vi "Soft_Robot_Model.vi"() -> ()   [LabVIEW 2015]
uses:
  <vilib>/addons/Control Design/_Stochastic Systems/Stochastic Systems.llb/Stochastic Systems SubVIs/cd_Stochastic State-Space Model.ctl
  <vilib>/addons/Control Design/_Model Construction/Model Typedefs.llb/CD State Space Model (MIMO).ctl
  <vilib>/addons/Control Design/_Model Construction/Model Typedefs.llb/CD General Elements.ctl
  <vilib>/addons/Control Design/_Stochastic Systems/Stochastic Systems.llb/Stochastic Systems SubVIs/cd_Second-Order Statistics Noise Model.ctl
  <vilib>/Analysis/Matrix/Datatypes/RealMatrix.ctl
  <vilib>/addons/Control Design/_Stochastic Systems/Stochastic Systems.llb/CD CtoD Stochastic Model.ctl
  <vilib>/Analysis/7linalg.llb/Eigenvalue and Vectors Output Option.ctl
  <vilib>/Platform/TimedLoop/XDataNode/timing_clust.ctl
  <vilib>/Platform/TimedLoop/XDataNode/nitl_modes.ctl
  <vilib>/Platform/TimedLoop/XDataNode/wakeup.ctl
  <vilib>/addons/Control Design/_Stochastic Systems/Stochastic Systems.llb/CD Construct Stochastic Model (Numeric).vi
  <vilib>/Analysis/7linalg.llb/Create Special Real Matrix.vi
  <vilib>/addons/Control Design/_Stochastic Systems/Stochastic Systems.llb/CD Construct Noise Model (Numeric).vi
  <vilib>/Analysis/7linalg.llb/Real Eigenvalues and Vectors.vi
  <vilib>/addons/Control Design/_State Feedback Control/State Feedback Control.llb/State Feedback Control SubVis/cd_Linear Quadratic Regulator.vi
  <vilib>/FPGAPlugInAG/myRIO-1900/niLvFpga_Open_myRIO-1900.vi
  <vilib>/rvi/interface/common/dynamic/niFpgaDynamicAddResources.vi
  <vilib>/Utility/error.llb/Error Cluster From Error Code.vi
  <vilib>/rvi/errors/niLvFpgaAdjustHostInterfaceError.vi
  <vilib>/FPGAPlugInAG/Dynamic/niLvFpga_Close_Dynamic.vi
  <vilib>/Utility/file.llb/Write Delimited Spreadsheet (DBL).vi
  <vilib>/Utility/file.llb/Write Delimited Spreadsheet (I64).vi
  <vilib>/addons/Control Design/_Time Response Analysis/Time Response.llb/Time Response subVI/cd_Impulse Response (State-Space).vi
  <vilib>/addons/Control Design/_Time Response Analysis/Time Response.llb/Time Response subVI/cd_Step Response (State-Space).vi
  <vilib>/Simulation/Estimation/Implementation/NILVSim Discrete Kalman Filter.llb/SIM Disc KF Pred and Corr with Pred Gain with Checking Direct LV.vi
  <vilib>/addons/Control Design/_Implementation/CD State Feedback Controller (Multiple Outputs).vi
  <vilib>/Platform/TimedLoop/XDataNode/XDataNode.xnode
  <vilib>/rvi/interface/nirviOpenFPGA/nirviOpenFPGA.xnode
  FPGA Bitfiles/ACC20115_FPGATarget_CurrentControlle_W-6n2rsGK8k.lvbitx
  Misc/Current Controller.vi
  <vilib>/rvi/interface/nirviReadWriteControl/nirviReadWriteControl.xnode
  <vilib>/rvi/interface/nirviCloseFPGA/nirviCloseFPGA.xnode
  <vilib>/Simulation/Implementation/XNodeFramework/SimXNode/SimX.xnode
  <vilib>/addons/Control Design/_State Feedback Control/NI_CD_State Feedback Control.lvlib
  <vilib>/Analysis/NI_AALPro.lvlib
  <vilib>/Platform/TimedLoop/XDataNode/XDNodeRunTimeDep.lvlib
  <vilib>/rvi/interface/Simulation/niFpgaSimulationCallBeginRW.vi
  <vilib>/addons/Control Design/_Stochastic Systems/NI_CD_Stochastic Systems.lvlib
  <vilib>/addons/Control Design/_State-Space Analysis/NI_CD_State-Space Analysis.lvlib
  <vilib>/addons/Control Design/_Implementation/NI_CD_Implementation.lvlib
  <vilib>/addons/Control Design/_Time Response Analysis/NI_CD_Time Response.lvlib
  NiFpgaLv.dll
  <vilib>/addons/Control Design/_Model Construction/NI_LinSys_Model Typedefs.lvlib
  <vilib>/Analysis/Matrix/NI_Matrix.lvlib
panel:
  in  "Tab Control":T1(tab)
  out "Valve Current (mA)":dbl(graph)=181.17310975569308
  out "Kinect Fusion":dbl(graph)=696.694
  in  "Current (mA)":i32
  out "KF Xhat(k|k)":dbl[][](graph)
  out "Plant Output and KF estimation":dbl[][](graph)=[[694.135, 693.2125685090368]]
  out "KF Predictor Gain L(k)":dbl[][](array[numeric])=[[1.0]] format="%#.6g"
  out "KF Gain M(k)":dbl[][](array[numeric]) format="%#.6g"
  in  "Stop":bool
  out "LQR Eigenvalues":cdb[](array[numeric]) format="%.5f"
  out "P(k+1|k)":dbl[][](array[numeric])
  out "P(k|k)":dbl[][](array[numeric])
  out "LQR Q Eig Vals":cdb[](array[numeric])
  out "LQR R Eig Val":cdb[](array[numeric])
  out "Optimal LQR Gains":dbl[][](array[numeric])
  out "Control Action":dbl
  out "Controllable?":bool
  out "Stable?":bool
  out "Detectable?":bool
  out "Observable?":bool
  out "LQR Q Matrix":T2
  out "LQR R Matrix":T2
  out "FPGA Overflow?":bool
  in  "Set Point (mm)":dbl(knob)=641.7660208643815 scale=680.0..700.0
  out "Stochastic SS Model":T3={"Sampling Time (s)"=0.0, "G"=[], "B"=[[-1.71e-07], [6.47e-07]], "A"=[], "C"=[], "D"=[], "H"=[]} {"H" format="%#.2g"; "D" format="%#.2g"; "C" format="%#.2g"; "A" format="%#.2g"; "B" format="%#.2g"; "G" format="%#.2g"; "Sampling Time (s)" format="%.2f"}
  out "Deterministic SS Model":T4={"properties"={"Model name"="", "Input names"=[], "Output names"=[], "Input Delays"=[], "Output Delays"=[], "Sampling Time"=0.0, "Notes"=""}, "A"=[], "B"=[[-1.706e-07], [6.469e-07]], "C"=[], "D"=[], "StateNames"=[], "Transport Delay"=[]} {"Transport Delay" format="%.2f"; "D" format="%#.2g"; "C" format="%#.2g"; "B" format="%#.2g"; "A" format="%#.2g"; "properties"."Sampling Time" format="%#.6p"; "properties"."Output Delays" format="%.4f"; "properties"."Input Delays" format="%.4f"}
  out "DAC Loop Error":errorcluster
  out "LQR Error":errorcluster
  out "KF Noise Model":T6 {"N" format="%#.2g"; "R" format="%#.2g"; "E{v}" format="%#.2g"; "E{w}" format="%#.2g"; "Q" format="%#.2g"}
  out "FPGA Loop Error":errorcluster
  out "Control Loop Error":errorcluster
  out "KF Model Error":errorcluster
  out "UDP Loop Error":errorcluster
  out "Step Response Graph":cluster{"time":dbl[], dbl[]}[](graph)=[{"time"=[0.0, 0.1, 0.2, 0.30000000000000004, 0.4, 0.5, 0.6000000000000001, 0.7000000000000001, 0.8, 0.9, 1.0, 1.1, 1.2000000000000002, 1.3, 1.4000000000000001, 1.5, 1.6, 1.7000000000000002, 1.8, 1.9000000000000001, 2.0, 2.1, 2.2, 2.3000000000000003, 2.4000000000000004, 2.5, 2.6, 2.7, 2.8000000000000003, 2.9000000000000004, 3.0, 3.1, 3.2, 3.3000000000000003, 3.4000000000000004, 3.5, 3.6, 3.7, 3.8000000000000003, 3.9000000000000004, 4.0, 4.1000000000000005, 4.2, 4.3, 4.4, 4.5, 4.6000000000000005, 4.7, 4.800000000000001, 4.9, 5.0, 5.1000000000000005, 5.2, 5.300000000000001, 5.4, 5.5, 5.6000000000000005, 5.7, 5.800000000000001, 5.9, 6.0, 6.1000000000000005, 6.2, 6.300000000000001, 6.4, 6.5, 6.6000000000000005, 6.7, 6.800000000000001, 6.9, 7.0, 7.1000000000000005, 7.2, 7.300000000000001, 7.4, 7.5, 7.6000000000000005, 7.7, 7.800000000000001, 7.9, 8.0], [0.0, 0.0004663473208612627, 0.0017296930483795164, 0.0035885524413313812, 0.00585108885158747, 0.008342022204108804, 0.010907538001557412, 0.013418337758795643, 0.01577103010603519, 0.017888100567384182, 0.019716719021094366, 0.02122664935211373, 0.022407518377011763, 0.02326568343598631, 0.02382091276348735, 0.024103062386256875, 0.024148900146291487, 0.023999193507947617, 0.02369614475738421, 0.023281226369499006, 0.02279344169187109, 0.022268012342287972, 0.021735474206151545, 0.021221148763839872, 0.020744945570676618, 0.020321444775591793, 0.01996020519209235, 0.019666243132932183, 0.01944062944497821, 0.019281156374667745, 0.019183031510994153, 0.01913956258079366, 0.019142803850451515, 0.019184141922185993, 0.01925480547445023, 0.01934628972900578, 0.019450691946355205, 0.019560958936806403, 0.019671051366119408, 0.01977603252338114, 0.019872091237783975, 0.01995650984687708, 0.020027588622327185, 0.02008453795668775, 0.020127349020610013, 0.02015665263024424, 0.020173574831124263, 0.02017959631108057, 0.02017642129264157, 0.02016586010332895, 0.020149728243942358, 0.02012976351919565, 0.020107561696361465, 0.0200845302370225, 0.0200618589138676, 0.02004050557782586, 0.020021194971562285, 0.020004428277976674, 0.01999050102686616, 0.019979527036564866, 0.0199714662161444, 0.019966154273690646, 0.019963332644441115, 0.019962677248304108, 0.019963824991160707, 0.019966397222957007, 0.019970019645588307, 0.019974338415697335, 0.019979032405429503, 0.019983821764274674, 0.01998847306610796, 0.01999280142814749, 0.019996670055101227, 0.019999987695808956, 0.020002704505559007, 0.020004806789810977, 0.02000631106930135, 0.020007257857379883, 0.020007705482562522, 0.0200077242268862, 0.02000739098734998]}]
  out "Impulse Response":cluster{"time":dbl[], dbl[]}[](graph)=[{"time"=[0.0, 0.1, 0.2, 0.30000000000000004, 0.4, 0.5, 0.6000000000000001, 0.7000000000000001, 0.8, 0.9, 1.0, 1.1, 1.2000000000000002, 1.3, 1.4000000000000001, 1.5, 1.6, 1.7000000000000002, 1.8, 1.9000000000000001, 2.0, 2.1, 2.2, 2.3000000000000003, 2.4000000000000004, 2.5, 2.6, 2.7, 2.8000000000000003, 2.9000000000000004, 3.0, 3.1, 3.2, 3.3000000000000003, 3.4000000000000004, 3.5, 3.6, 3.7, 3.8000000000000003, 3.9000000000000004, 4.0, 4.1000000000000005, 4.2, 4.3, 4.4, 4.5, 4.6000000000000005, 4.7, 4.800000000000001, 4.9, 5.0, 5.1000000000000005, 5.2, 5.300000000000001, 5.4, 5.5, 5.6000000000000005, 5.7, 5.800000000000001, 5.9, 6.0, 6.1000000000000005, 6.2, 6.300000000000001, 6.4, 6.5, 6.6000000000000005, 6.7, 6.800000000000001, 6.9, 7.0, 7.1000000000000005, 7.2, 7.300000000000001, 7.4, 7.5, 7.6000000000000005, 7.7, 7.800000000000001, 7.9, 8.0], [0.0, 0.008988172215977587, 0.015941438633037666, 0.02091487162309135, 0.024042908393783827, 0.02551889757722494, 0.02557569478365717, 0.024467992676866855, 0.022456868580669295, 0.019796844996257237, 0.016725591461953054, 0.013456253705261323, 0.010172280017081137, 0.007024525658691236, 0.004130353039235721, 0.0015744064999214857, -0.0005892768149515742, -0.002334157452931432, -0.0036574068645988137, -0.004575736995437892, -0.005121104002831364, -0.005336502802076594, -0.005272025764550862, -0.004981315552097141, -0.004518500722641401, -0.003935664888301879, -0.0032808669235171064, -0.0025967016806585676, -0.001919368189106927, -0.0012781953978247278, -0.0006955639255905182, -0.0001871555662120171, 0.0002375401230830873, 0.0005745316131444697, 0.0008245089129275849, 0.0009919638112413014, 0.0010842980213564997, 0.0011109616697939839, 0.0010826555079039139, 0.0010106212985917036, 0.0009060364188353945, 0.0007795211078167689, 0.000640760178844977, 0.0004982355180431294, 0.00035906135961267507, 0.00022891114129368586, 0.0001120226402826769, 1.1266967989904443e-05, -7.17332656671379e-05, -0.00013645086398689086, -0.0001832792705777772, -0.0002133479298936649, -0.00022833790229576505, -0.0002303060085980187, -0.00022152389413133484, -0.00020433657074322872, -0.00018104328983030286, -0.0001538020745465803, -0.00012455793086593947, -9.499368500849999e-05, -6.650156442132397e-05, -4.0173044664881016e-05, -1.6804109357439747e-05, 3.087108111676786e-06, 1.9233341685522883e-05, 3.158477953815003e-05, 4.027189426429472e-05, 4.556687476968165e-05, 4.7845653868121716e-05, 4.755213725597536e-05, 4.516584913005334e-05, 4.117383523520003e-05, 3.6047319585871326e-05, 3.0223306623967816e-05, 2.4091062632339335e-05, 1.7983202024296476e-05, 1.2170946052935176e-05, 6.863011578249593e-06, 2.207522022942255e-06, -1.7036935523276584e-06, -4.8290401595337954e-06]}]
  out "Step and Impulse Response Plots":cluster{"time":dbl[], dbl[]}[](graph)=[{"time"=[0.0, 0.1, 0.2, 0.30000000000000004, 0.4, 0.5, 0.6000000000000001, 0.7000000000000001, 0.8, 0.9, 1.0, 1.1, 1.2000000000000002, 1.3, 1.4000000000000001, 1.5, 1.6, 1.7000000000000002, 1.8, 1.9000000000000001, 2.0, 2.1, 2.2, 2.3000000000000003, 2.4000000000000004, 2.5, 2.6, 2.7, 2.8000000000000003, 2.9000000000000004, 3.0, 3.1, 3.2, 3.3000000000000003, 3.4000000000000004, 3.5, 3.6, 3.7, 3.8000000000000003, 3.9000000000000004, 4.0, 4.1000000000000005, 4.2, 4.3, 4.4, 4.5, 4.6000000000000005, 4.7, 4.800000000000001, 4.9, 5.0, 5.1000000000000005, 5.2, 5.300000000000001, 5.4, 5.5, 5.6000000000000005, 5.7, 5.800000000000001, 5.9, 6.0, 6.1000000000000005, 6.2, 6.300000000000001, 6.4, 6.5, 6.6000000000000005, 6.7, 6.800000000000001, 6.9, 7.0, 7.1000000000000005, 7.2, 7.300000000000001, 7.4, 7.5, 7.6000000000000005, 7.7, 7.800000000000001, 7.9, 8.0], [0.0, 0.0004663473208612627, 0.0017296930483795164, 0.0035885524413313812, 0.00585108885158747, 0.008342022204108804, 0.010907538001557412, 0.013418337758795643, 0.01577103010603519, 0.017888100567384182, 0.019716719021094366, 0.02122664935211373, 0.022407518377011763, 0.02326568343598631, 0.02382091276348735, 0.024103062386256875, 0.024148900146291487, 0.023999193507947617, 0.02369614475738421, 0.023281226369499006, 0.02279344169187109, 0.022268012342287972, 0.021735474206151545, 0.021221148763839872, 0.020744945570676618, 0.020321444775591793, 0.01996020519209235, 0.019666243132932183, 0.01944062944497821, 0.019281156374667745, 0.019183031510994153, 0.01913956258079366, 0.019142803850451515, 0.019184141922185993, 0.01925480547445023, 0.01934628972900578, 0.019450691946355205, 0.019560958936806403, 0.019671051366119408, 0.01977603252338114, 0.019872091237783975, 0.01995650984687708, 0.020027588622327185, 0.02008453795668775, 0.020127349020610013, 0.02015665263024424, 0.020173574831124263, 0.02017959631108057, 0.02017642129264157, 0.02016586010332895, 0.020149728243942358, 0.02012976351919565, 0.020107561696361465, 0.0200845302370225, 0.0200618589138676, 0.02004050557782586, 0.020021194971562285, 0.020004428277976674, 0.01999050102686616, 0.019979527036564866, 0.0199714662161444, 0.019966154273690646, 0.019963332644441115, 0.019962677248304108, 0.019963824991160707, 0.019966397222957007, 0.019970019645588307, 0.019974338415697335, 0.019979032405429503, 0.019983821764274674, 0.01998847306610796, 0.01999280142814749, 0.019996670055101227, 0.019999987695808956, 0.020002704505559007, 0.020004806789810977, 0.02000631106930135, 0.020007257857379883, 0.020007705482562522, 0.0200077242268862, 0.02000739098734998]}, {"time"=[0.0, 0.1, 0.2, 0.30000000000000004, 0.4, 0.5, 0.6000000000000001, 0.7000000000000001, 0.8, 0.9, 1.0, 1.1, 1.2000000000000002, 1.3, 1.4000000000000001, 1.5, 1.6, 1.7000000000000002, 1.8, 1.9000000000000001, 2.0, 2.1, 2.2, 2.3000000000000003, 2.4000000000000004, 2.5, 2.6, 2.7, 2.8000000000000003, 2.9000000000000004, 3.0, 3.1, 3.2, 3.3000000000000003, 3.4000000000000004, 3.5, 3.6, 3.7, 3.8000000000000003, 3.9000000000000004, 4.0, 4.1000000000000005, 4.2, 4.3, 4.4, 4.5, 4.6000000000000005, 4.7, 4.800000000000001, 4.9, 5.0, 5.1000000000000005, 5.2, 5.300000000000001, 5.4, 5.5, 5.6000000000000005, 5.7, 5.800000000000001, 5.9, 6.0, 6.1000000000000005, 6.2, 6.300000000000001, 6.4, 6.5, 6.6000000000000005, 6.7, 6.800000000000001, 6.9, 7.0, 7.1000000000000005, 7.2, 7.300000000000001, 7.4, 7.5, 7.6000000000000005, 7.7, 7.800000000000001, 7.9, 8.0], [0.0, 0.008988172215977587, 0.015941438633037666, 0.02091487162309135, 0.024042908393783827, 0.02551889757722494, 0.02557569478365717, 0.024467992676866855, 0.022456868580669295, 0.019796844996257237, 0.016725591461953054, 0.013456253705261323, 0.010172280017081137, 0.007024525658691236, 0.004130353039235721, 0.0015744064999214857, -0.0005892768149515742, -0.002334157452931432, -0.0036574068645988137, -0.004575736995437892, -0.005121104002831364, -0.005336502802076594, -0.005272025764550862, -0.004981315552097141, -0.004518500722641401, -0.003935664888301879, -0.0032808669235171064, -0.0025967016806585676, -0.001919368189106927, -0.0012781953978247278, -0.0006955639255905182, -0.0001871555662120171, 0.0002375401230830873, 0.0005745316131444697, 0.0008245089129275849, 0.0009919638112413014, 0.0010842980213564997, 0.0011109616697939839, 0.0010826555079039139, 0.0010106212985917036, 0.0009060364188353945, 0.0007795211078167689, 0.000640760178844977, 0.0004982355180431294, 0.00035906135961267507, 0.00022891114129368586, 0.0001120226402826769, 1.1266967989904443e-05, -7.17332656671379e-05, -0.00013645086398689086, -0.0001832792705777772, -0.0002133479298936649, -0.00022833790229576505, -0.0002303060085980187, -0.00022152389413133484, -0.00020433657074322872, -0.00018104328983030286, -0.0001538020745465803, -0.00012455793086593947, -9.499368500849999e-05, -6.650156442132397e-05, -4.0173044664881016e-05, -1.6804109357439747e-05, 3.087108111676786e-06, 1.9233341685522883e-05, 3.158477953815003e-05, 4.027189426429472e-05, 4.556687476968165e-05, 4.7845653868121716e-05, 4.755213725597536e-05, 4.516584913005334e-05, 4.117383523520003e-05, 3.6047319585871326e-05, 3.0223306623967816e-05, 2.4091062632339335e-05, 1.7983202024296476e-05, 1.2170946052935176e-05, 6.863011578249593e-06, 2.207522022942255e-06, -1.7036935523276584e-06, -4.8290401595337954e-06]}]
  in  "A":dbl[][](array[numeric])=[[-0.275, -0.05848], [0.3155, 0.05955]] format="%#.5g"
  in  "B":dbl[][](array[numeric])=[[-0.0001629], [8.009e-05]] format="%#.5g"
  in  "C":dbl[][](array[numeric])=[[0.742, 2.316]] format="%#.5g"
  in  "G":dbl[][](array[numeric])=[[0.7998], [2.296]] format="%#.2g"
  in  "xhat(0|-1)":dbl[](array[numeric])=[687.0, 687.0]
  in  "P(0|-1)":dbl[][](array[numeric])=[[1.0, 0.0], [0.0, 1.0]]
  in  "LQR Matrix (Q)":dbl[](array[slide])=[1.5199110829529336, 8.111308307896874] scale=0.01..1000000.0
  in  "LQR R":dbl[](array[slide])=[0.8629156295881086] scale=0.1..10.0
  in  "KF R":dbl[](array[slide])=[0.013076604860118303] scale=0.001..5000.0
  in  "KF Q":dbl[](array[slide])=[0.44512793318037663] scale=0.01..100.0
  in  "yhat(KT)":path=path "c:/SRS.csv"
  in  "input":path
  in  "y(kT)":path=path "c:/SRS.csv"
  in  "SP":path
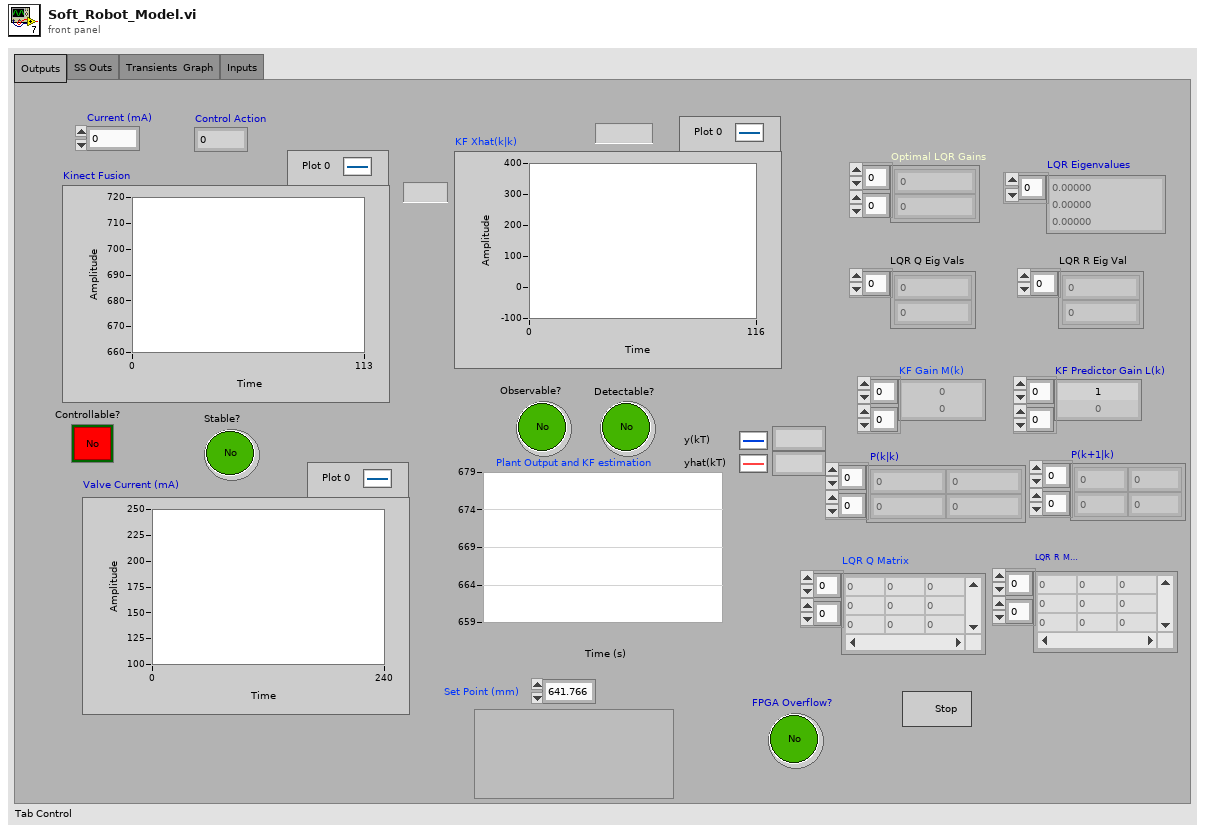
[diagram p1: front panel]
types:
  T1 = enum32{"Outputs", "SS Outs", "Transients  Graph", "Inputs"}
  T2 = typedef "NI_Matrix.lvlib/RealMatrix.ctl" = dbl[][]
  T3 = typedef "NI_CD_Stochastic Systems.lvlib/cd_Stochastic State-Space Model.ctl" = cluster{"Sampling Time (s)":dbl, "G":dbl[][], "B":dbl[][], "A":dbl[][], "C":dbl[][], "D":dbl[][], "H":dbl[][]}
  T4 = typedef "NI_LinSys_Model Typedefs.lvlib/CD State Space Model (MIMO).ctl" = cluster{"properties":T5, "A":dbl[][], "B":dbl[][], "C":dbl[][], "D":dbl[][], "StateNames":string[], "Transport Delay":dbl[][]}
  T5 = typedef "NI_LinSys_Model Typedefs.lvlib/CD General Elements.ctl" = cluster{"Model name":string, "Input names":string[], "Output names":string[], "Input Delays":dbl[], "Output Delays":dbl[], "Sampling Time":dbl, "Notes":string}
  T6 = typedef "NI_CD_Stochastic Systems.lvlib/cd_Second-Order Statistics Noise Model.ctl" = cluster{"Q":dbl[][], "E{w}":dbl[], "E{v}":dbl[], "R":dbl[][], "N":dbl[][]}
  T7 = typedef "NI_AALPro.lvlib/Eigenvalue and Vectors Output Option.ctl" = i32
  T8 = enum32{"Identity", "Diagonal", "Toepliz", "Vandermonde", "Companion"}
  T9 = typedef "NI_CD_Stochastic Systems.lvlib/CD CtoD Stochastic Model.ctl" = enum16{"Truncation of Taylor Series", "Numerical Integration"}
  T10 = enum16{"state weighting", "output weighting, Dim Q = Ny", "output weighting, Dim Q = Nx"}
  T11 = typedef "XDNodeRunTimeDep.lvlib/timing_clust.ctl" = cluster{"Expected End [f-1]":u64, "Actual End [f-1]":u64, "Finished Late? [f-1]":bool, "Expected End [i-1]":u64, "Actual End [i-1]":u64, "Finished Late? [i-1]":bool, "Expected Start [i]":u64, "Actual Start [i]":u64, "Expected Start [f]":u64, "Actual Start [f]":u64, "Source Name":string, "Structure Name":string, "Period":i64, "Deadline":i64, "Offset":i64, "Start":i64, "Priority":i32, "Timeout":i32, "Mode":T12, "Wakeup Reason":T13, "Error":errorcluster, "Source Type":string, "Secondary Source Type":string, "Global End Time":u64, "Global Start Time":u64, "Frame Duration":u64, "Iteration Duration":u64, "Assigned CPU":i32, "I/O Scan Engine Mode":u32}
  T12 = typedef "XDNodeRunTimeDep.lvlib/nitl_modes.ctl" = enum32{"No Change", "Process missed periods, maintain original phase", "Discard missed periods, maintain original phase", "Process missed periods, ignore original phase", "Discard missed periods, ignore original phase"}
  T13 = typedef "XDNodeRunTimeDep.lvlib/wakeup.ctl" = enum32{"Normal", "Aborted", "Asynchronous wakeup", "Timing source error", "Timed loop error", "Timeout"}
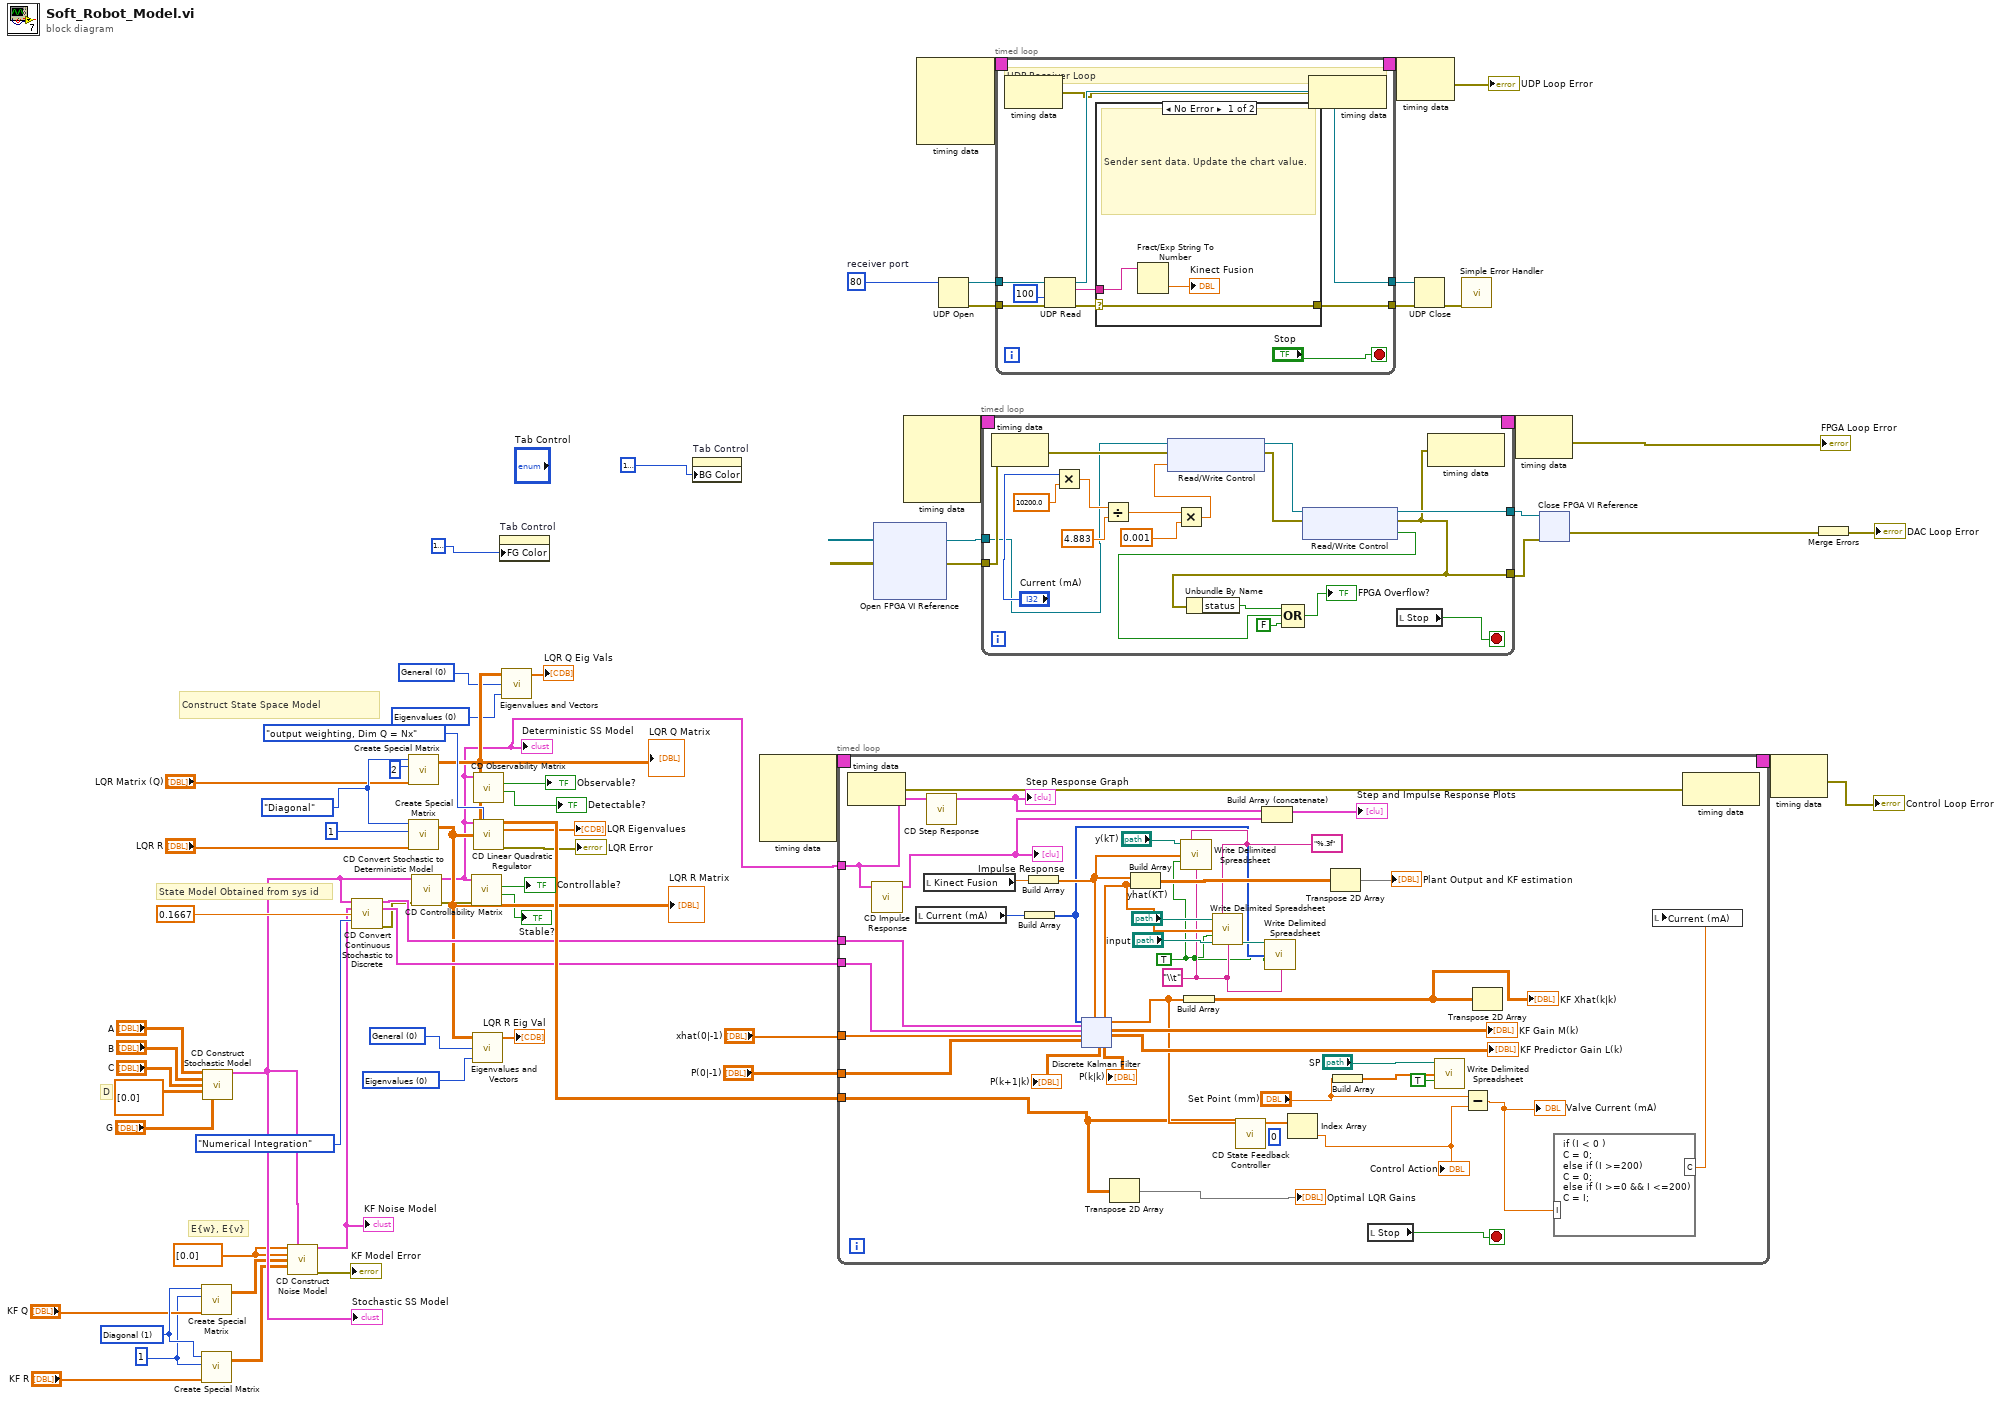
[diagram p0: block diagram]
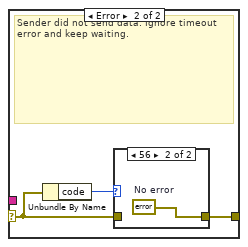
[diagram p2: hidden frame]
diagram:
  w10 = T7 0 items=["Eigenvalues", "Eigenvalues & Vectors"] ("output option")
  w11 = 0 items=["General", "Symmetric"] ("matrix type")
  w13 = T7 0 items=["Eigenvalues", "Eigenvalues & Vectors"] ("output option")
  w14 = 0 items=["General", "Symmetric"] ("matrix type")
  w20 = T8."Diagonal" ("matrix type")
  w21 = 1 ("KF Q/R Size")
  w25 = dbl[] [0.0] ("E{w}")
  w26 = 1 items=["Identity", "Diagonal", "Toeplitz", "Vandermonde", "Companion", "Hankel", "Hadamard", "Wilkinson", "Hilbert", "Inverse Hilbert", "Rosser", "Pascal"] ("matrix type")
  w56 = u16 80  # receiver port
  # "E{w}, E{v}"
  # "D"
  # "State Model Obtained from sys id"
  # "Construct State Space Model"
  n1 = call-poly <vilib>:"Create Special Matrix.vi"("matrix type"=w26, "matrix size"=w21, "Input Vector1"="KF Q") -> ("Special Matrix"=w28:T2)  [unwired: 2 in, 1 out]
  n2 = call-poly <vilib>:"Create Special Matrix.vi"("matrix type"=w26, "matrix size"=w21, "Input Vector1"="KF R") -> ("Special Matrix"=w27:T2)  [unwired: 2 in, 1 out]
  n3 = call-poly <vilib>:"CD Construct Stochastic Model.vi"("A"="A", "B"="B", "C"="C", "D"=dbl[][] [[0.0]], "G"="G") -> ("Stochastic State-Space Model"=w35:T3)  [unwired: 3 in, 7 out]
  "Stochastic SS Model" <- w35
  n4 = call-poly <vilib>:"CD Construct Noise Model.vi"("E{w}"=w25, "Stochastic State-Space Model"=w35, "E{v}"=w25, "Q"=w28, "R"=w27) -> ("Second-Order Statistics Noise Model out"=w36:T6, "error out"=→"KF Model Error":errorcluster)  [unwired: 2 in, 7 out]
  "KF Noise Model" <- w36
  n5 = call <vilib>:"CD Convert Continuous Stochastic to Discrete.vi"("Continuous Stochastic\nState-Space Model"=w35, "Continuous Second-Order\nStatistics Noise Model"=w36, "Sampling Time (s)"=0.1667, "Method"=CD_CtoD_Stochastic_Model."Numerical Integration") -> ("Discrete Stochastic\nState-Space Model"=w45:T3, "Discrete Second-Order\nStatistics Noise Model"=w46:T6, "error out"=w34:errorcluster)  [unwired: 1 in, 8 out]
  n6 = call-poly <vilib>:"Create Special Matrix.vi"("matrix type"=w20, "matrix size"=2, "Input Vector1"="LQR Matrix (Q)") -> ("Special Matrix"=w15:T2)  [unwired: 2 in, 1 out]
  "LQR Q Matrix" <- w15
  n7 = call-poly <vilib>:"Create Special Matrix.vi"("matrix type"=w20, "matrix size"=1, "Input Vector1"="LQR R") -> ("Special Matrix"=w8:T2)  [unwired: 2 in, 1 out]
  "LQR R Matrix" <- w8
  n8 = call <vilib>:"CD Convert Stochastic to Deterministic Model.vi"("Stochastic State-Space Model"=w35, "error in (no error)"=w34) -> ("Deterministic State-Space Model"=w3:T4, "error out"=w33:errorcluster)  [unwired: 12 in]
  "Deterministic SS Model" <- w3
  n9 = call <vilib>:"CD Controllability Matrix.vi"("error in (no error)"=w33, "State-Space Model"=w3) -> ("Is Stabilizable?"=→"Stable?":bool, "Is Controllable?"=→"Controllable?":bool)  [unwired: 6 in, 2 out]
  n10 = call-poly <vilib>:"Eigenvalues and Vectors.vi"("output option"=w10, "matrix type"=w11, "Input Matrix"=w8) -> ("Eigenvalues"=→"LQR R Eig Val":cdb[])  [unwired: 2 out]
  n11 = call <vilib>:"CD Observability Matrix.vi"("State-Space Model"=w3) -> ("Is Detectable?"=→"Detectable?":bool, "Is Observable?"=→"Observable?":bool)  [unwired: 7 in, 2 out]
  n12 = call-poly <vilib>:"CD Linear Quadratic Regulator.vi"("State-Space Model"=w3, "Weighting Type"=T10."output weighting, Dim Q = Nx", "Q"=w15, "R"=w8) -> ("Optimal Gain (K)"=w47:dbl[][], "Eigenvalues"=→"LQR Eigenvalues":cdb[], "error out"=→"LQR Error":errorcluster)  [unwired: 8 in, 1 out]
  n13 = property on="Tab Control" class="TabCtl (strict)"("FG Color"=u32 16777226) -> ()  [unwired: 2 in, 2 out]
  n14 = call-poly <vilib>:"Eigenvalues and Vectors.vi"("output option"=w13, "matrix type"=w14, "Input Matrix"=w15) -> ("Eigenvalues"=→"LQR Q Eig Vals":cdb[])  [unwired: 2 out]
  n15 = property on="Tab Control" class="TabCtl (strict)"("BG Color"=u32 16777226) -> ()  [unwired: 2 in, 2 out]
  n16 = node-c288() -> (w49:T11)  [unwired: 4 in]
  n17 = timed-loop {
    timing: w49 -> [_]
    timing-out: [_] -> w48
    tunnel: w47 -> [w92]
    tunnel: w46 -> [w107]
    tunnel: w45 -> [w97]
    tunnel: "xhat(0|-1)" -> [w106]
    tunnel: "P(0|-1)" -> [w105]
    tunnel: w3 -> [w90]
    stop <- w94 stop-if-true
    w79 = "\\t" ("delimiter (\\t)")
    w70 = TRUE ("transpose? (F)")
    w78 = "%.3f" ("format (%.3f)")
    (unwired) 0 ("index")
    n18 = node-c288() -> (w98:errorcluster)  [unwired: 1 in]
    n19 = call-poly <vilib>:"CD Impulse Response.vi"("State-Space Model"=w90) -> ("Impulse Response Graph"=w88:cluster{"time":dbl[], dbl[]}[])  [unwired: 7 in, 3 out]
    "Impulse Response" <- w88
    n20 = local read "Current (mA)"() -> (w99:i32)
    n21 = local read "Kinect Fusion"() -> (w100:dbl)
    n22 = call-poly <vilib>:"CD Step Response.vi"("State-Space Model"=w90) -> ("Step Response Graph"=w87:cluster{"time":dbl[], dbl[]}[])  [unwired: 7 in, 3 out]
    "Step Response Graph" <- w87
    n23 = Build Array ("Build Array 5")(w99) -> (w75:i32[])
    n24 = Build Array ("Build Array 3")(w100) -> (w76:dbl[])
    n25 = xnode ("Discrete Kalman Filter")("input u(k)"=w75, "Stochastic State-Space Model"=w97, "Second-Order Statistics Noise Model"=w107, "Initial State Estimate xhat(0|-1)"=w106, "Initial Estimation Error Covariance P(0|-1)"=w105, "Output y(k)"=w76) -> ("Prediction Error Covariance P(k+1|k)"=→"P(k+1|k)":dbl[][], "Estimated Output yhat(k)"=w80:dbl[], "Filter Error Covariance P(k|k)"=→"P(k|k)":dbl[][], "Corrected State Estimate xhat(k|k)"=w101:dbl[], "Kalman Filter Gain M(k)"=→"KF Gain M(k)":dbl[][], "Kalman Predictor Gain L(k)"=→"KF Predictor Gain L(k)":dbl[][])  [unwired: 2 in, 2 out]
    n26 = Transpose 2D Array(2D array=w92) -> (transposed array=→"Optimal LQR Gains":dbl[][])
    n27 = Build Array(w76, w80) -> (w86:dbl[][])
    n28 = call-poly <vilib>:"Write Delimited Spreadsheet.vi"("file path (dialog if empty)"="y(kT)", "format (%.3f)"=w78, "1D data"=w76, "append to file? (F)"=w70, "delimiter (\\t)"=w79) -> ()  [unwired: 9 in, 2 out]
    n29 = Build Array ("Build Array 2")(w101) -> (w69:dbl[][])
    "KF Xhat(k|k)" <- w69
    n30 = call-poly <vilib>:"Write Delimited Spreadsheet.vi"("file path (dialog if empty)"="yhat(KT)", "format (%.3f)"=w78, "1D data"=w80, "append to file? (F)"=w70, "delimiter (\\t)"=w79) -> ()  [unwired: 9 in, 2 out]
    n31 = call-poly <vilib>:"CD State Feedback Controller.vi"("Controller Gain"=w92, "States"=w101) -> ("Controller Action"=w104:dbl[])  [unwired: 8 in, 1 out]
    n32 = Build Array (concatenate)(w87, w88) -> (→"Step and Impulse Response Plots":cluster{"time":dbl[], dbl[]}[])
    n33 = call-poly <vilib>:"Write Delimited Spreadsheet.vi"("file path (dialog if empty)"="input", "1D data"=w75, "append to file? (F)"=w70, "delimiter (\\t)"=w79) -> ()  [unwired: 10 in, 2 out]
    n34 = Index Array(array=w104) -> (element=w91:dbl)  [unwired: 1 in]
    "Control Action" <- w91
    n35 = Transpose 2D Array(2D array=w86) -> (transposed array=→"Plant Output and KF estimation":dbl[][])
    n36 = Build Array("Set Point (mm)") -> (w73:dbl[])
    n37 = local read "Stop"() -> (w94:bool)
    n38 = call-poly <vilib>:"Write Delimited Spreadsheet.vi"("file path (dialog if empty)"="SP", "1D data"=w73, "append to file? (F)"=TRUE) -> ()  [unwired: 11 in, 2 out]
    n39 = Subtract ("Subtract 2")(x="Set Point (mm)", y=w91) -> (x-y=w84:dbl)
    "Valve Current (mA)" <- w84
    n40 = Transpose 2D Array(2D array=w69) -> ()  [unwired: 1 out]
    n41 = formula code="if (I < 0 )\nC = 0;\nelse if (I >=200)\nC = 0;\nelse if (I >=0 && I <=200)\nC = I;"("I"=w84) -> ("C"=w83:dbl)
    n42 = local write "Current (mA)"(w83) -> ()
    n43 = node-c288(w98) -> ()  [unwired: 1 out]
  }
  n44 = xnode "Open FPGA VI Reference"() -> ("FPGA VI Reference Out"=w55:refnum<k20>, "error out"=w54:errorcluster)  [unwired: 2 in]
  n45 = node-c288() -> (w66:T11)  [unwired: 4 in]
  n46 = node-c288() -> (w53:T11)  [unwired: 4 in]
  n47 = UDP Open(11:w56) -> (port=w57:refnum<k16>, 0:w58:errorcluster)  [unwired: 4 in, 1 out]
  n48 = timed-loop {
    tunnel: w54 -> [w133]
    tunnel: [w132] -> w64
    tunnel: [w141] -> w68
    timing: w66 -> [_]
    timing-out: [_] -> w65
    tunnel: w55 -> [w131]
    stop <- w130 stop-if-true
    n49 = node-c288() -> ()  [unwired: 1 in, 1 out]
    n50 = Multiply(x="Current (mA)", y=10200.0) -> (x*y=w136:dbl)
    n51 = Divide(x=w136, y=4.883) -> (x/y=w139:dbl)
    n52 = Multiply(x=w139, y=0.001) -> (x*y=w135:dbl)
    n53 = xnode "Read/Write Control"("FPGA VI Reference In"=w131, "error in"=w133, "DAC Inlet Valve"=w135) -> ("FPGA VI Reference Out"=w146:refnum<k20>, "error out"=w145:errorcluster)
    n54 = xnode "Read/Write Control"("FPGA VI Reference In"=w146, "error in"=w145) -> ("FPGA VI Reference Out"=w141:refnum<k20>, "error out"=w132:errorcluster, "Inlet Overflow?"=w142:bool)
    n55 = Unbundle By Name(w132) -> ("status"=w143:bool)
    n56 = Compound Arithmetic op=OR(w143, w142, FALSE ("value")) -> (→"FPGA Overflow?":bool)
    n57 = local read "Stop"() -> (w130:bool)
    n58 = node-c288(w132) -> ()  [unwired: 1 out]
  }
  n59 = timed-loop {
    tunnel: w57 -> [w159]
    tunnel: [w153] -> w61
    tunnel: w58 -> [w158]
    tunnel: [w154] -> w59
    timing: w53 -> [_]
    timing-out: [_] -> w52
    stop <- "Stop" stop-if-true
    # "UDP Receiver Loop"
    n60 = node-c288() -> (w151:errorcluster)  [unwired: 1 in]
    n61 = UDP Read(connection ID=w159, timeout ms (25000)=100, 8:w158) -> (data out=w156:string, error out=w155:errorcluster, 3:w153:refnum<k16>)  [unwired: 3 out]
    n62 = case shown="No Error" w155 {
      selector: w155 -> [w165 w169]
      tunnel: w156 -> [w167 _]
      tunnel: [w165 w168] -> w154
      frame No Error {
        # "Sender sent data. Update the chart value."
        n63 = Fract/Exp String To Number(string=w167) -> (number=→"Kinect Fusion":dbl)  [unwired: 3 in, 1 out]
      }
      frame Error {
        # "Sender did not send data. Ignore timeout error and keep waiting."
        n64 = Unbundle By Name(w169) -> ("code"=w170:i32)
        n65 = case shown="56" w170 {
          tunnel: w169 -> [w171 _]
          tunnel: [w171 w172] -> w168
          frame Default {
          }
          frame 56 {
            w172 = errorcluster {"status"=FALSE, "code"=0, "source"=""}  # No error
          }
        }
      }
    }
    n66 = node-c288(w151) -> ()  [unwired: 1 out]
  }
  n67 = node-c288(w52) -> (→"UDP Loop Error":errorcluster)
  n68 = UDP Close(connection ID=w61, 8:w59) -> (error out=w60:errorcluster)  [unwired: 1 out]
  n69 = call <vilib>:"Simple Error Handler.vi"("error in (no error)"=w60) -> ()  [unwired: 1 in, 8 out]
  n70 = node-c288(w65) -> (→"FPGA Loop Error":errorcluster)
  n71 = xnode "Close FPGA VI Reference"("FPGA VI Reference In"=w68, "error in"=w64) -> ("error out"=w63:errorcluster)
  n72 = node-c288(w48) -> (→"Control Loop Error":errorcluster)
  n73 = Merge Errors(w63) -> (→"DAC Loop Error":errorcluster)
